vi "Main.vi"() -> ()   [LabVIEW 2014, in "teststand-api.lvlib" / "teststand-api.lvclass"]
uses:
  teststand-api.lvclass
  Model Run Mode--enum.ctl
  teststand-api.lvclass/teststand-api.ctl
panel:
  out "Shutdown":bool
  in  "Start":bool
  in  "stop":bool
  in  "Tab Control":enum32{"Page 1", "Page 2"}(tab)
  in  "Exec View":refnum<k7>(container)
  in  "Sequence View":refnum<k7>(container)
  in  "ExecutionView Manager":refnum<k7>(container)
  in  "SequenceFileView Manager":refnum<k7>(container)
  in  "App Manager":refnum<k7>(container)
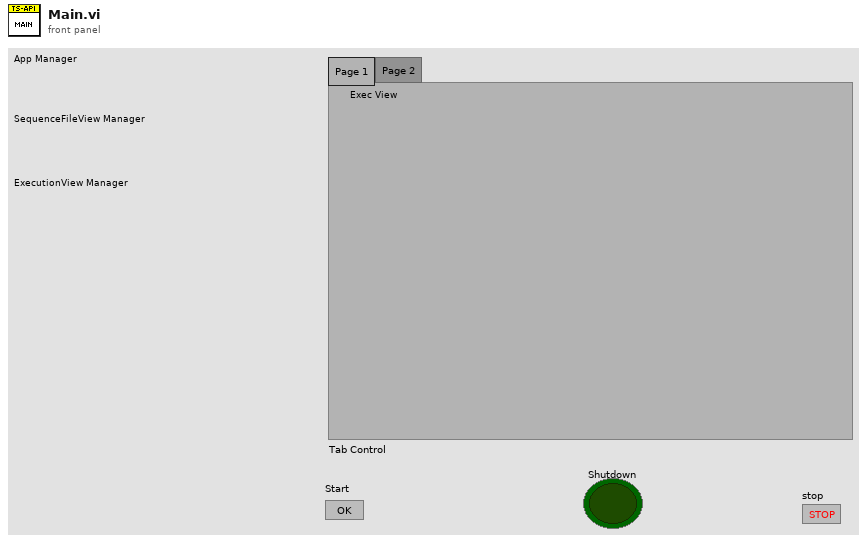
[diagram p1: front panel]
types:
  T1 = typedef "teststand-api.lvlib/teststand-api.lvclass/Model Run Mode--enum.ctl" = enum16{"Test UUTs", "Single Pass"}
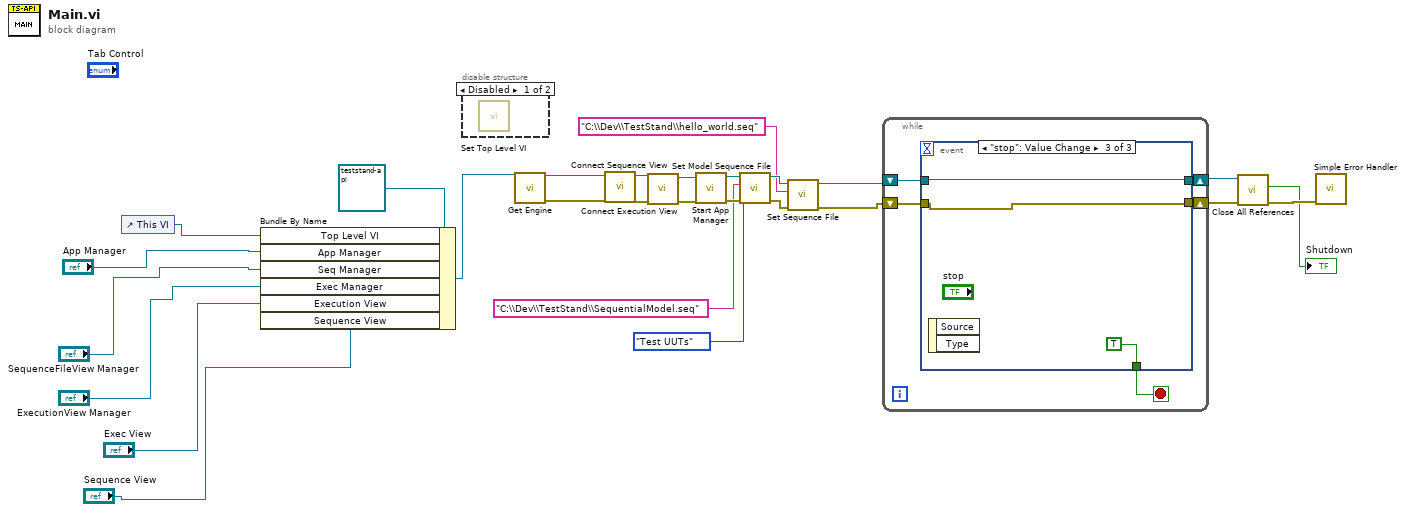
[diagram p0: block diagram]
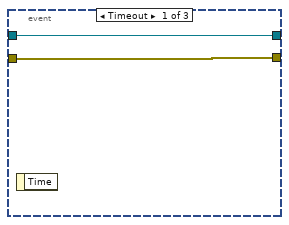
[diagram p3: hidden frame]
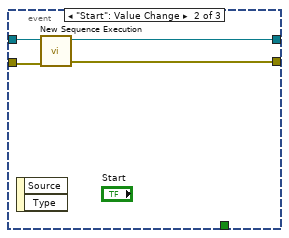
[diagram p4: hidden frame]
diagram:
  n1 = control-ref of="This VI"() -> (w4:refnum<vi>)
  n2 = Bundle By Name(cluster=refnum<class "teststand-api.lvclass"> refnum ("TestStand api in"), "Top Level VI"=w4, "App Manager"="App Manager", "Seq Manager"="SequenceFileView Manager", "Exec Manager"="ExecutionView Manager", "Execution View"="Exec View", "Sequence View"="Sequence View") -> (w19:refnum<class "teststand-api.lvclass">)
  n3 = disable-structure shown="Disabled" {
    frame Disabled {
      n4 = call-dynamic "Set Top Level VI.vi"() -> ()  [unwired: 10 in, 2 out]
    }
    frame Enabled {
    }
  }
  n5 = call-dynamic "Get Engine.vi"("ts-api in"=w19) -> ("error out"=w2:errorcluster, "ts-api out"=w3:refnum<class "teststand-api.lvclass">)  [unwired: 9 in]
  n6 = call-dynamic "Connect Sequence View.vi"("error in (no error)"=w2, "teststand-api in"=w3) -> ("error out"=w27:errorcluster, "teststand-api out"=w26:refnum<class "teststand-api.lvclass">)  [unwired: 8 in]
  n7 = call-dynamic "Connect Execution View.vi"("error in (no error)"=w27, "teststand-api in"=w26) -> ("error out"=w17:errorcluster, "teststand-api out"=w18:refnum<class "teststand-api.lvclass">)  [unwired: 8 in]
  n8 = call-dynamic "Start App Manager.vi"("error in (no error)"=w17, "teststand-api in"=w18) -> ("error out"=w15:errorcluster, "teststand-api out"=w16:refnum<class "teststand-api.lvclass">)  [unwired: 8 in]
  n9 = call-dynamic "Set Model Sequence File.vi"("error in (no error)"=w15, "Seq Model Run Mode"=Model_Run_Mode--enum."Test UUTs", "Model Seq File Path"="C:\\Dev\\TestStand\\SequentialModel.seq" ("ModelPath"), "teststand-api in"=w16) -> ("error out"=w14:errorcluster, "teststand-api out"=w13:refnum<class "teststand-api.lvclass">)  [unwired: 6 in]
  n10 = call-dynamic "Set Sequence File.vi"("error in (no error)"=w14, "Seq File Path"="C:\\Dev\\TestStand\\hello_world.seq" ("sequenceFilePath"), "teststand-api in"=w13) -> ("error out"=w8:errorcluster, "teststand-api out"=w9:refnum<class "teststand-api.lvclass">)  [unwired: 7 in]
  n11 = while {
    shift-right: [w31] -> w7
    shift-left: w9 -> [w32]
    shift-right: [w29] -> w6
    shift-left: w8 -> [w30]
    stop <- w28 stop-if-true
    n12 = event shown="[2] \"stop\": Value Change" {
      selector: _ -> [_ _ _]
      dyn-events: _ -> [_ _ _]
      timeout: _ -> [_ _ _]
      tunnel: w32 -> [w34 w38 w41]
      tunnel: [w34 w37 w41] -> w31
      tunnel: w30 -> [w33 w35 w40]
      tunnel: [w33 w36 w40] -> w29
      tunnel: [_ _ TRUE] -> w28
      event Timeout {
        n13 = event-data() -> ()  [unwired: 1 in, 1 out]
      }
      event "Start": Value Change {
        n14 = event-data() -> ()  [unwired: 1 in, 2 out]
        n15 = call-dynamic "New Sequence Execution.vi"("error in (no error)"=w35, "teststand-api in"=w38) -> ("error out"=w36:errorcluster, "teststand-api out"=w37:refnum<class "teststand-api.lvclass">)  [unwired: 8 in]
      }
      event "stop": Value Change {
        n16 = event-data() -> ()  [unwired: 1 in, 2 out]
      }
    }
  }
  n17 = call-dynamic "Close All References.vi"("error in (no error)"=w6, "teststand-api in"=w7) -> ("error out"=w5:errorcluster, "Shutdown"=→"Shutdown":bool)  [unwired: 7 in, 1 out]
  n18 = call <vilib>:"Simple Error Handler.vi"("error in (no error)"=w5) -> ()  [unwired: 4 in, 5 out]
